vi "HumidityDelay.vi"(8 "error in (no error)":errorcluster, 9 "Start Humidity":dbl=10.0 format="%#_13g", 11 "ArduinoControl in":refnum<class "ArduinoControl.lvclass">) -> (0 "error out":errorcluster, 3 "ArduinoControl out":refnum<class "ArduinoControl.lvclass">)   [LabVIEW 2019]
uses:
  ArduinoControl.lvclass
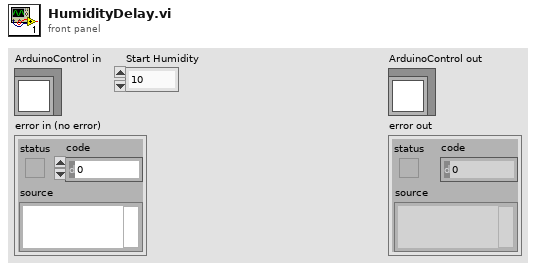
[diagram p1: front panel]
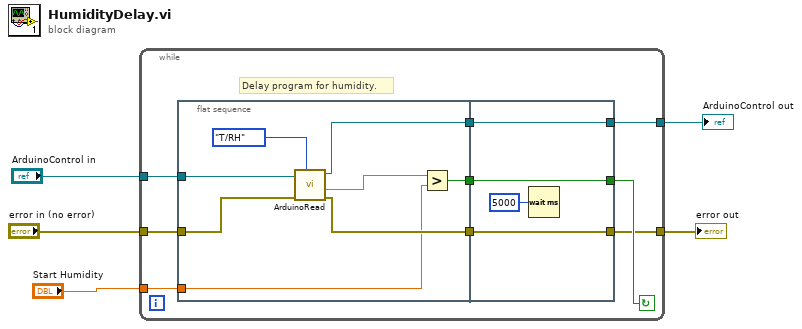
[diagram p0: block diagram]
diagram:
  n1 = while {
    tunnel: "ArduinoControl in" -> [w14]
    tunnel: "error in (no error)" -> [w13]
    tunnel: [w11] -> w3
    tunnel: [w10] -> w2
    tunnel: "Start Humidity" -> [w9]
    stop <- w12 continue-if-true
    # "Delay program for humidity."
    n2 = flat-sequence {
      tunnel: w14 -> [w22]
      tunnel: w13 -> [w19]
      tunnel: w9 -> [w15]
      tunnel: [w18] -> w8
      tunnel: [w17] -> w7
      tunnel: [w16] -> w6
      tunnel: [w24] -> w10
      tunnel: [w25] -> w11
      tunnel: [w26] -> w12
      tunnel: w8 -> [w26]
      tunnel: w7 -> [w25]
      tunnel: w6 -> [w24]
      frame #0 {
        n3 = call "ArduinoRead.vi"("Arduino function"=enum16{"T/RH", "Interlock", "Edgesense"}."T/RH", "error in (no error)"=w19, "ArduinoControl in"=w22) -> ("error out"=w16:errorcluster, "rel. Humidity [%]"=w20:dbl, "ArduinoControl out"=w17:refnum<class "ArduinoControl.lvclass">)  [unwired: 3 in, 3 out]
        n4 = Greater?(x=w20, y=w15) -> (0:w18:bool)
      }
      frame #1 {
        n5 = Wait (ms)(milliseconds to wait=u32 5000) -> ()  [unwired: 1 out]
      }
    }
  }
  "ArduinoControl out" <- w3
  "error out" <- w2
